vi "LV_UDP_client.vi"() -> ()   [LabVIEW 2020]
panel:
  in  "Send Test Image":bool
  in  "h":i32=10 min=1 max=5000 step=1
  in  "w":i32=1 min=1 max=5000 step=1
  out "Elaps ms":u32
  in  "Send Image":bool
  out "Path to Python script":path
  in  "Stop":bool
  out "Answer":string
  in  "Ping":bool
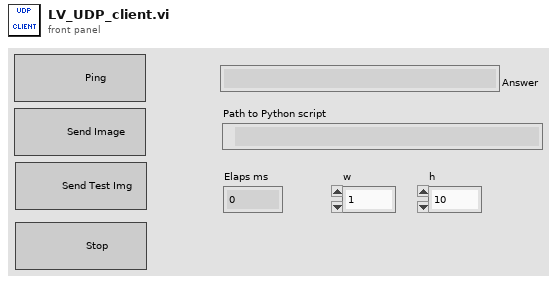
[diagram p1: front panel]
types:
  T1 = enum8{"Enabled", "Disabled", "Disabled and Grayed Out"}
  T2 = typedef "Image Type" = u32
  T3 = typedef "IMAQ Image.ctl" = refnum<image>
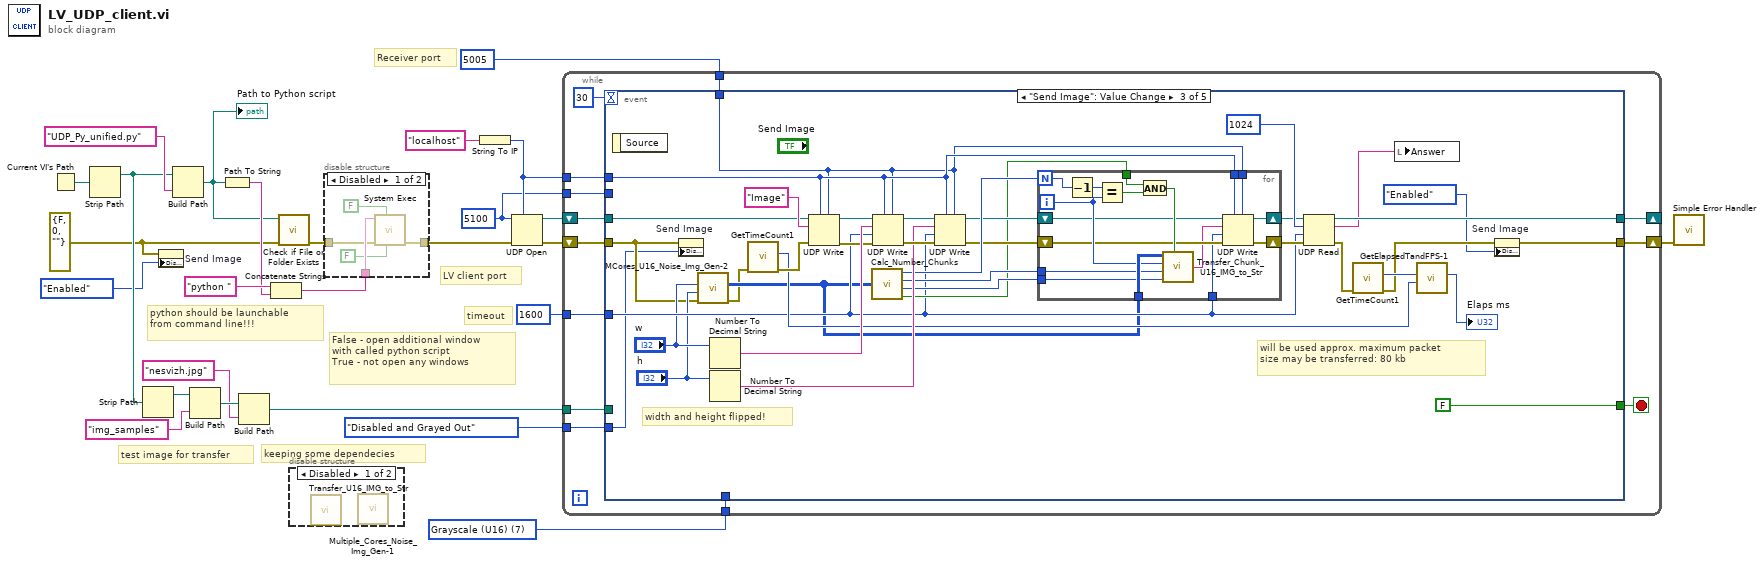
[diagram p0: block diagram]
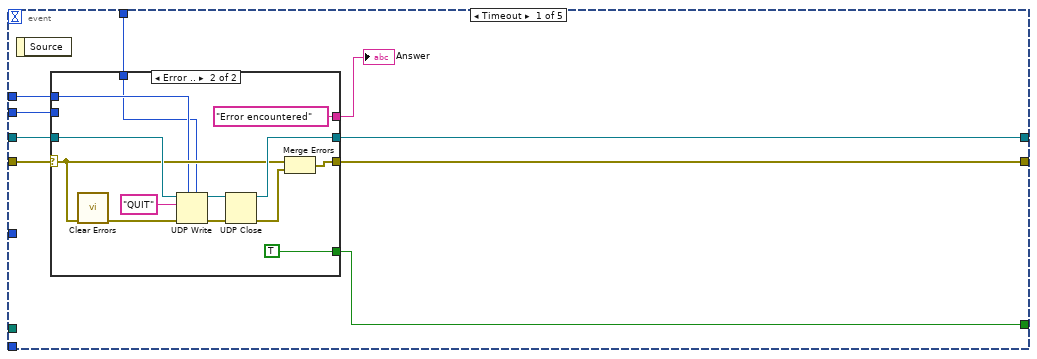
[diagram p4: hidden frame]
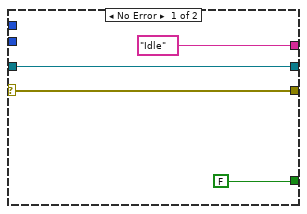
[diagram p5: hidden frame]
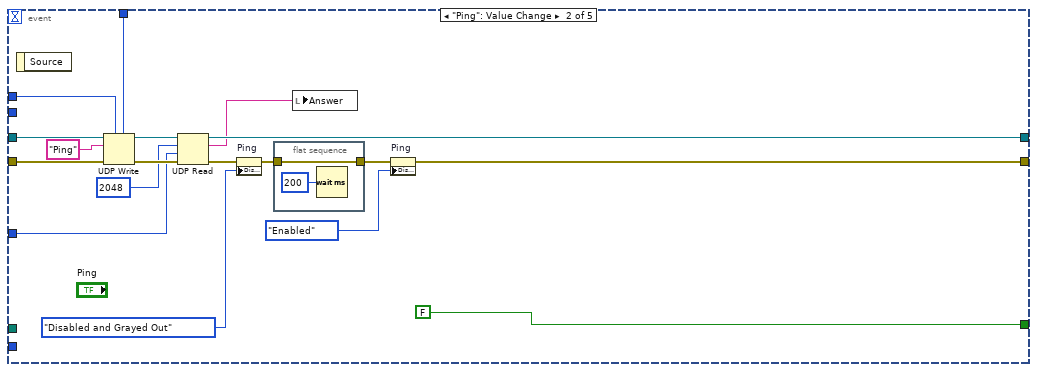
[diagram p6: hidden frame]
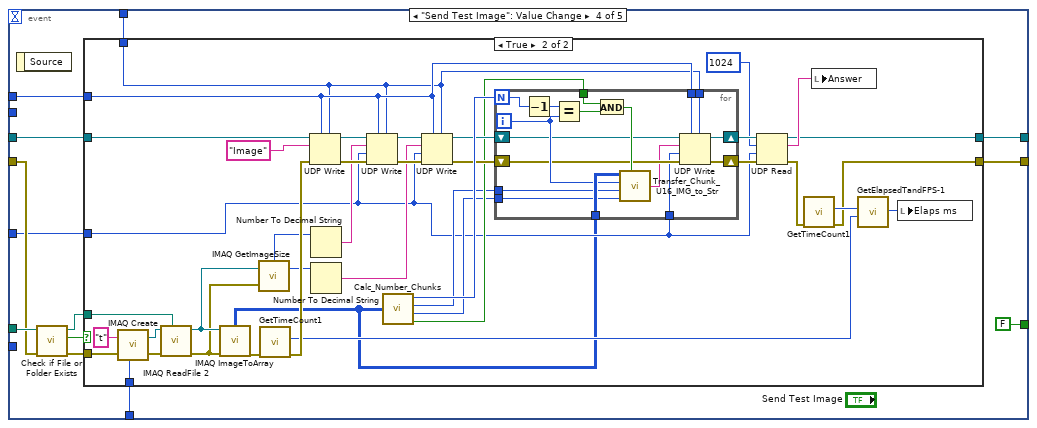
[diagram p7: hidden frame]
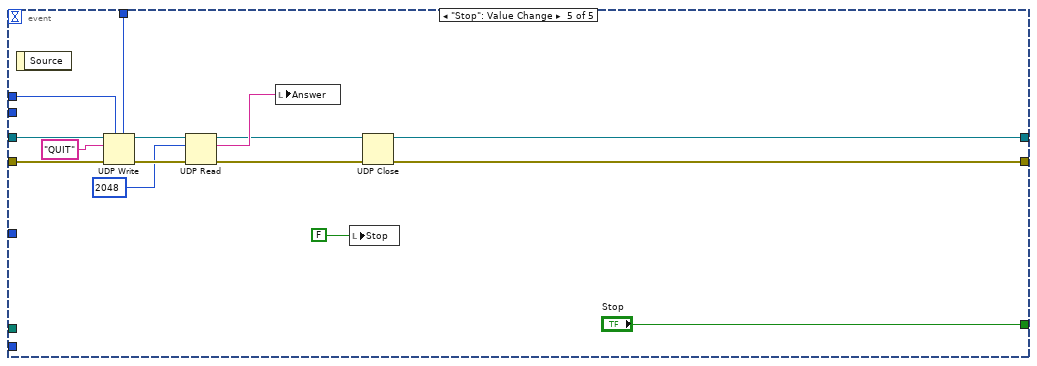
[diagram p9: hidden frame]
diagram:
  w4 = T2 7 items=["Grayscale (U8)", "Grayscale (I16)", "Grayscale (SGL)", "Complex (CSG)", "RGB (U32)", "HSL (U32)", "RGB (U64)", "Grayscale (U16)"] ("Image Type")
  w13 = u16 5100 ("remote port or service name")
  w2 = errorcluster {"status"=FALSE, "code"=0, "source"=""} ("error in (no error)")
  # "test image for transfer"
  # "keeping some dependecies"
  # "timeout"
  # "Receiver port"
  # "LV client port"
  # "False - open additional window\nwith called python script\nTrue - not open any windows"
  # "python should be launchable \nfrom command line!!!"
  n1 = Current VI's Path() -> (path=w25:path)
  n2 = Strip Path(path=w25) -> (stripped path=w10:path)  [unwired: 1 out]
  n3 = Strip Path(path=w10) -> (stripped path=w9:path)  [unwired: 1 out]
  n4 = property on="Send Image" class="Bool"(error in=w2, "DisabledEnum"=T1."Enabled" ("Disabled")) -> ()  [unwired: 1 in, 2 out]
  n5 = Build Path(base path=w10, name or relative path="UDP_Py_unified.py" ("string")) -> (appended path=w20:path)
  "Path to Python script" <- w20
  n6 = Build Path(base path=w9, name or relative path="img_samples" ("string")) -> (appended path=w7:path)
  n7 = Path To String(path=w20) -> (string=w21:string)
  n8 = Build Path(base path=w7, name or relative path="nesvizh.jpg" ("string")) -> (appended path=w5:path)
  n9 = Concatenate Strings("python " ("command line"), w21) -> (w23:string)
  n10 = call <vilib>:"Check if File or Folder Exists.vi"("error in (no error)"=w2, "path"=w20) -> ("error out"=w19:errorcluster)  [unwired: 7 in, 2 out]
  n11 = disable-structure shown="Disabled" {
    frame Disabled {
      n12 = call "Transfer_U16_IMG_to_Str.vi"() -> ()  [unwired: 1 in, 1 out]
      n13 = call "Multiple_Cores_Noise_Img_Gen-1.vi"() -> ()  [unwired: 10 in, 2 out]
    }
    frame Enabled {
    }
  }
  n14 = disable-structure shown="Disabled" {
    disable-tunnel: w23 -> [w31 _]
    disable-tunnel: [w30 w32] -> w18
    disable-tunnel: w19 -> [w28 w32]
    frame Disabled {
      n15 = call <vilib>:"System Exec.vi"("run minimized? (F)"=FALSE, "wait until completion? (T)"=FALSE, "error in (no error)"=w28, "command line"=w31) -> ("error out"=w30:errorcluster)  [unwired: 4 in, 3 out]
    }
    frame Enabled {
    }
  }
  n16 = String To IP(1:"localhost" ("address")) -> (0:w14:u32)
  n17 = UDP Open(7:w14, 8:w18, 11:w13) -> (port=w16:refnum<k16>, 0:w17:errorcluster)  [unwired: 2 in, 1 out]
  n18 = while {
    shift-right: [w42] -> _
    shift-left: w16 -> [w43]
    shift-right: [w40] -> w26
    shift-left: w17 -> [w44]
    tunnel: w14 -> [w38]
    tunnel: w13 -> [w39]
    tunnel: u16 5005 ("remote port or service name") -> [w37]
    tunnel: 1600 -> [w36]
    tunnel: w5 -> [w35]
    tunnel: w4 -> [w34]
    tunnel: T1."Disabled and Grayed Out" ("Disabled") -> [w33]
    stop <- w41 stop-if-true
    n19 = event shown="[2] \"Send Image\": Value Change" {
      selector: _ -> [_ _ _ _ _]
      dyn-events: _ -> [_ _ _ _ _]
      timeout: 30 -> [_ _ _ _ _]
      tunnel: [w50 FALSE ("Stop") FALSE ("Stop") FALSE ("Stop") "Stop"] -> w41
      tunnel: w44 -> [w54 w83 w96 w156 w227]
      tunnel: w43 -> [w53 w82 w127 w151 w228]
      tunnel: [w52 w78 w121 w146 w229] -> w42
      tunnel: [w51 w85 w93 w147 w230] -> w40
      tunnel: w39 -> [w48 _ _ _ _]
      tunnel: w38 -> [w47 w74 w102 w150 w219]
      tunnel: w37 -> [w46 w73 w101 w149 w218]
      tunnel: w36 -> [_ w72 w103 w148 _]
      tunnel: w35 -> [_ _ _ w157 _]
      tunnel: w34 -> [_ _ _ w152 _]
      tunnel: w33 -> [_ _ w95 _ _]
      event Timeout {
        n20 = event-data() -> ()  [unwired: 1 in, 1 out]
        n21 = case shown="Error .." w54 {
          selector: w54 -> [w57 w62]
          tunnel: [w58 w69] -> w52
          tunnel: w53 -> [w58 w68]
          tunnel: [w57 w63] -> w51
          tunnel: [FALSE ("Stop") TRUE ("Stop")] -> w50
          tunnel: ["Idle" ("Answer") "Error encountered" ("Answer")] -> w49
          tunnel: w48 -> [_ _]
          tunnel: w47 -> [_ w60]
          tunnel: w46 -> [_ w59]
          frame No Error {
          }
          frame Error {
            n22 = call <vilib>:"Clear Errors.vi"("error in (no error)"=w62) -> ("error out"=w67:errorcluster)  [unwired: 5 in, 1 out]
            n23 = UDP Write(address=w60, port or service name=w59, connection ID=w68, data in="QUIT", 8:w67) -> (error out=w66:errorcluster, 3:w64:refnum<k16>)  [unwired: 1 in]
            n24 = UDP Close(connection ID=w64, 8:w66) -> (connection ID out=w69:refnum<k16>, error out=w61:errorcluster)
            n25 = Merge Errors(w62, w61) -> (w63:errorcluster)
          }
        }
        "Answer" <- w49
      }
      event "Ping": Value Change {
        n26 = event-data() -> ()  [unwired: 1 in, 1 out]
        n27 = UDP Write(address=w74, port or service name=w73, connection ID=w82, data in="Ping", 8:w83) -> (error out=w80:errorcluster, 3:w79:refnum<k16>)  [unwired: 1 in]
        n28 = UDP Read(connection ID=w79, max size (548)=2048 ("bytes to read"), timeout ms (25000)=w72, 8:w80) -> (data out=w75:string, error out=w77:errorcluster, 3:w78:refnum<k16>)  [unwired: 2 out]
        n29 = property on="Ping" class="Bool"(error in=w77, "DisabledEnum"=T1."Disabled and Grayed Out" ("Disabled")) -> (error out=w88:errorcluster)  [unwired: 1 in, 1 out]
        n30 = flat-sequence {
          tunnel: w88 -> [w90]
          tunnel: [w90] -> w86
          frame #0 {
            n31 = Wait (ms)(milliseconds to wait=u32 200) -> ()  [unwired: 1 out]
          }
        }
        n32 = local write "Answer"(w75) -> ()
        n33 = property on="Ping" class="Bool"(error in=w86, "DisabledEnum"=T1."Enabled" ("Disabled")) -> (error out=w85:errorcluster)  [unwired: 1 in, 1 out]
      }
      event "Send Image": Value Change {
        # "width and height flipped!"
        # "will be used approx. maximum packet \nsize may be transferred: 80 kb"
        n34 = event-data() -> ()  [unwired: 1 in, 1 out]
        n35 = property on="Send Image" class="Bool"(error in=w96, "DisabledEnum"=w95) -> ()  [unwired: 1 in, 2 out]
        n36 = call "MCores_U16_Noise_Img_Gen-2.vi"("error IN"=w96, "[IN] Width"="h", "[IN] Height"="w") -> ("error OUT"=w99:errorcluster, "[OUT] U16 Pixel Img"=w100:u16[][])  [unwired: 7 in]
        n37 = Number To Decimal String(number="w") -> (decimal integer string=w123:string)  [unwired: 1 in]
        n38 = Number To Decimal String(number="h") -> (decimal integer string=w119:string)  [unwired: 1 in]
        n39 = call "GetTimeCount1.vi"("error IN"=w99) -> ("error OUT"=w116:errorcluster, "[OUT] Timer Count"=w113:u32)  [unwired: 9 in]
        n40 = UDP Write(address=w102, port or service name=w101, connection ID=w127, data in="Image", 8:w116) -> (error out=w117:errorcluster, 3:w118:refnum<k16>)  [unwired: 1 in]
        n41 = call "Calc_Number_Chunks.vi"("[IN] U16 Pixel Img"=w100) -> ("[OUT] Number of chunks"=w110:i32, "[OUT] # rows single transfer"=w109:i32, "[OUT] # rows last transfer"=w108:i32, "[OUT] Not-equal last transfer"=w104:bool)
        n42 = UDP Write(address=w102, port or service name=w101, connection ID=w118, data in=w123, 8:w117, 9:w103) -> (error out=w126:errorcluster, 3:w125:refnum<k16>)
        n43 = UDP Write(address=w102, port or service name=w101, connection ID=w125, data in=w119, 8:w126, 9:w103) -> (error out=w106:errorcluster, 3:w107:refnum<k16>)
        n44 = for {
          N: w110 -> [w145]
          shift-right: [w135] -> w111
          shift-left: w106 -> [w136]
          tunnel: w100 -> [w143]
          tunnel: w109 -> [w138]
          tunnel: w108 -> [w137]
          shift-right: [w134] -> w105
          shift-left: w107 -> [w133]
          tunnel: w104 -> [w140]
          tunnel: w103 -> [w131]
          tunnel: w102 -> [w130]
          tunnel: w101 -> [w129]
          i -> [w141]
          n45 = Decrement(x=w145) -> (x-1=w144:i32)
          n46 = Equal?(x=w144, y=w141) -> (x = y?=w139:bool)
          n47 = And(x=w140, y=w139) -> (x .and. y?=w142:bool)
          n48 = call "Transfer_Chunk_U16_IMG_to_Str.vi"("[IN] U16 Pixel Img"=w143, "[IN] # of chunk"=w141, "[IN] # rows single transfer"=w138, "[IN] # rows last transfer"=w137, "[IN] Use remained rows"=w142) -> ("[OUT] Converted String"=w132:string)
          n49 = UDP Write(address=w130, port or service name=w129, connection ID=w133, data in=w132, 8:w136, 9:w131) -> (error out=w135:errorcluster, 3:w134:refnum<k16>)
        }
        n50 = UDP Read(connection ID=w105, max size (548)=1024 ("bytes to read"), timeout ms (25000)=w103, 8:w111) -> (data out=w120:string, error out=w115:errorcluster, 3:w121:refnum<k16>)  [unwired: 2 out]
        n51 = call "GetTimeCount1.vi"("error IN"=w115) -> ("error OUT"=w94:errorcluster, "[OUT] Timer Count"=w114:u32)  [unwired: 9 in]
        n52 = local write "Answer"(w120) -> ()
        n53 = call "GetElapsedTandFPS-1.vi"("[IN] Timer Count Before ALL [ms]"=w113, "[IN] Timer Count After ALL [ms]"=w114) -> ("[OUT] Elapsed time [ms]"=→"Elaps ms":u32)  [unwired: 3 in, 2 out]
        n54 = property on="Send Image" class="Bool"(error in=w94, "DisabledEnum"=T1."Enabled" ("Disabled")) -> (error out=w93:errorcluster)  [unwired: 1 in, 1 out]
      }
      event "Send Test Image": Value Change {
        n55 = event-data() -> ()  [unwired: 1 in, 1 out]
        n56 = call <vilib>:"Check if File or Folder Exists.vi"("error in (no error)"=w156, "path"=w157) -> ("error out"=w155:errorcluster, "file or folder exists?"=w154:bool, "dup path"=w153:path)  [unwired: 7 in]
        n57 = case shown="True" w154 {
          tunnel: w155 -> [w159 w200]
          tunnel: w153 -> [_ w195]
          tunnel: w152 -> [_ w199]
          tunnel: w151 -> [w160 w193]
          tunnel: w150 -> [_ w174]
          tunnel: w149 -> [_ w173]
          tunnel: w148 -> [_ w170]
          tunnel: [w159 w163] -> w147
          tunnel: [w160 w162] -> w146
          frame False {
          }
          frame True {
            n58 = call "IMAQ Create"("Image Name"="t", "Image Type"=w199, "error in (no error)"=w200) -> ("New Image"=w196:T3, "error out"=w197:errorcluster)  [unwired: 2 in]
            n59 = call "IMAQ ReadFile 2"("File Path"=w195, "error in (no error)"=w197, "Image"=w196) -> ("error out"=w189:errorcluster, "Image Out"=w190:T3)  [unwired: 4 in, 3 out]
            n60 = call "IMAQ ImageToArray"("error in (no error)"=w189, "Image"=w190) -> ("error out"=w194:errorcluster, "Image Pixels (U8)"=w161:u8[][])  [unwired: 2 in, 3 out]
            n61 = call "IMAQ GetImageSize"("Image"=w190, "error in (no error)"=w189) -> ("Y Resolution"=w187:i32, "X Resolution"=w188:i32)  [unwired: 2 in, 1 out]
            n62 = call "GetTimeCount1.vi"("error IN"=w194) -> ("error OUT"=w192:errorcluster, "[OUT] Timer Count"=w166:u32)  [unwired: 9 in]
            n63 = UDP Write(address=w174, port or service name=w173, connection ID=w193, data in="Image", 8:w192) -> (error out=w186:errorcluster, 3:w185:refnum<k16>)  [unwired: 1 in]
            n64 = Number To Decimal String(number=w188) -> (decimal integer string=w184:string)  [unwired: 1 in]
            n65 = Number To Decimal String(number=w187) -> (decimal integer string=w181:string)  [unwired: 1 in]
            n66 = UDP Write(address=w174, port or service name=w173, connection ID=w185, data in=w184, 8:w186, 9:w170) -> (error out=w182:errorcluster, 3:w183:refnum<k16>)
            n67 = call "Calc_Number_Chunks.vi"("[IN] U16 Pixel Img"=w161) -> ("[OUT] Number of chunks"=w180:i32, "[OUT] # rows single transfer"=w176:i32, "[OUT] # rows last transfer"=w175:i32, "[OUT] Not-equal last transfer"=w177:bool)
            n68 = UDP Write(address=w174, port or service name=w173, connection ID=w183, data in=w181, 8:w182, 9:w170) -> (error out=w178:errorcluster, 3:w179:refnum<k16>)
            n69 = for {
              N: w180 -> [w217]
              shift-right: [w207] -> w172
              shift-left: w178 -> [w208]
              tunnel: w161 -> [w215]
              tunnel: w176 -> [w210]
              tunnel: w175 -> [w209]
              shift-right: [w206] -> w171
              shift-left: w179 -> [w205]
              tunnel: w177 -> [w212]
              tunnel: w170 -> [w203]
              tunnel: w174 -> [w202]
              tunnel: w173 -> [w201]
              i -> [w213]
              n70 = Decrement(x=w217) -> (x-1=w216:i32)
              n71 = Equal?(x=w216, y=w213) -> (x = y?=w211:bool)
              n72 = And(x=w212, y=w211) -> (x .and. y?=w214:bool)
              n73 = call "Transfer_Chunk_U16_IMG_to_Str.vi"("[IN] U16 Pixel Img"=w215, "[IN] # of chunk"=w213, "[IN] # rows single transfer"=w210, "[IN] # rows last transfer"=w209, "[IN] Use remained rows"=w214) -> ("[OUT] Converted String"=w204:string)
              n74 = UDP Write(address=w202, port or service name=w201, connection ID=w205, data in=w204, 8:w208, 9:w203) -> (error out=w207:errorcluster, 3:w206:refnum<k16>)
            }
            n75 = UDP Read(connection ID=w171, max size (548)=1024 ("bytes to read"), timeout ms (25000)=w170, 8:w172) -> (data out=w169:string, error out=w168:errorcluster, 3:w162:refnum<k16>)  [unwired: 2 out]
            n76 = call "GetTimeCount1.vi"("error IN"=w168) -> ("error OUT"=w163:errorcluster, "[OUT] Timer Count"=w167:u32)  [unwired: 9 in]
            n77 = local write "Answer"(w169) -> ()
            n78 = call "GetElapsedTandFPS-1.vi"("[IN] Timer Count Before ALL [ms]"=w166, "[IN] Timer Count After ALL [ms]"=w167) -> ("[OUT] Elapsed time [ms]"=w164:u32)  [unwired: 3 in, 2 out]
            n79 = local write "Elaps ms"(w164) -> ()
          }
        }
      }
      event "Stop": Value Change {
        n80 = event-data() -> ()  [unwired: 1 in, 1 out]
        n81 = UDP Write(address=w219, port or service name=w218, connection ID=w228, data in="QUIT", 8:w227) -> (error out=w224:errorcluster, 3:w225:refnum<k16>)  [unwired: 1 in]
        n82 = UDP Read(connection ID=w225, max size (548)=2048 ("bytes to read"), 8:w224) -> (data out=w222:string, error out=w223:errorcluster, 3:w221:refnum<k16>)  [unwired: 1 in, 2 out]
        n83 = local write "Answer"(w222) -> ()
        n84 = local write "Stop"(FALSE ("Stop")) -> ()
        n85 = UDP Close(connection ID=w221, 8:w223) -> (connection ID out=w229:refnum<k16>, error out=w230:errorcluster)
      }
    }
  }
  n86 = call <vilib>:"Simple Error Handler.vi"("error in (no error)"=w26) -> ()  [unwired: 4 in, 5 out]
